vi "Define Sweep Segments Table.vi"(0 "VISA resource name":refnum<visa-resource-name>, 1 "Stimulus Mode (0: Start/Stop)":u16(ring) items=["Start/Stop", "Center/Span"], 2 "Number of Segments (1)":i32=1, 3 "Start/Center (0)":dbl[](array[numeric]), 4 "Stop/Span (0)":dbl[](array[numeric]), 5 "error in (no error)":errorcluster, 6 "Channel (1)":i32=1, 7 "Measurement Points (0)":dbl[](array[numeric]), 8 "Sweep Mode  (0)":dbl[](array[numeric]), 9 "IF Bandwidth (0)":dbl[](array[numeric]), 10 "Sweep Time (F: Disable)":bool, 11 "Power  (0)":dbl[](array[numeric]), 12 "Sweep Time  (0)":dbl[](array[numeric]), 13 "Sweep Delay Time  (0)":dbl[](array[numeric])) -> (14 "VISA resource name out":refnum<visa-resource-name>, 19 "error out":errorcluster)   [LabVIEW 2018, in "Agilent ENA Series.lvlib"]
doc: "Loads the sweep segments into instrument."
uses:
  Agilent ENA Series.lvlib
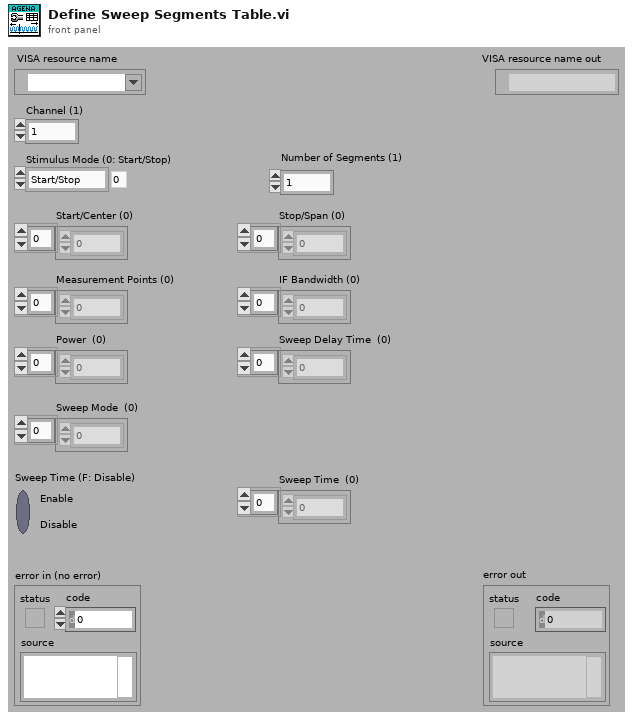
[diagram p1: front panel]
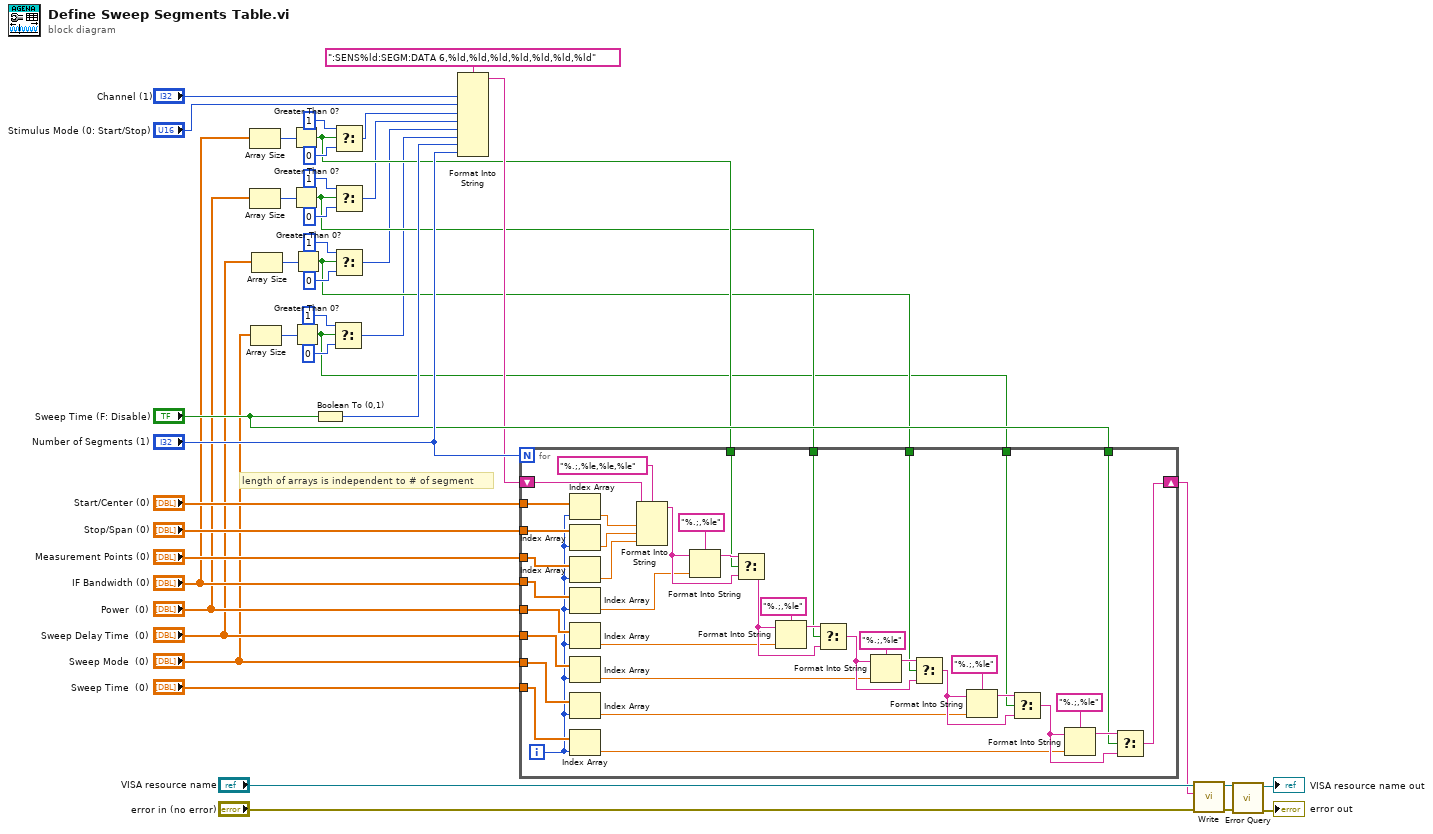
[diagram p0: block diagram]
diagram:
  # "length of arrays is independent to # of segment"
  n1 = Array Size(array="IF Bandwidth (0)") -> (size(s)=w21:i32)
  n2 = Array Size(array="Power  (0)") -> (size(s)=w18:i32)
  n3 = Array Size(array="Sweep Mode  (0)") -> (size(s)=w6:i32)
  n4 = Array Size(array="Sweep Delay Time  (0)") -> (size(s)=w10:i32)
  n5 = Greater Than 0?(x=w21) -> (x > 0?=w20:bool)
  n6 = Greater Than 0?(x=w18) -> (x > 0?=w15:bool)
  n7 = Greater Than 0?(x=w6) -> (x > 0?=w2:bool)
  n8 = Greater Than 0?(x=w10) -> (x > 0?=w9:bool)
  n9 = Boolean To (0,1)(Boolean="Sweep Time (F: Disable)") -> (0, 1=w37:i16)
  n10 = Select(t=1, s=w2, f=0) -> (s? t:f=w3:i32)
  n11 = Select(t=1, s=w20, f=0) -> (s? t:f=w19:i32)
  n12 = Select(t=1, s=w15, f=0) -> (s? t:f=w14:i32)
  n13 = Select(t=1, s=w9, f=0) -> (s? t:f=w8:i32)
  n14 = Format Into String(format string=":SENS%ld:SEGM:DATA 6,%ld,%ld,%ld,%ld,%ld,%ld,%ld", "Channel (1)", "Stimulus Mode (0: Start/Stop)", w19, w14, w8, w3, w37, "Number of Segments (1)") -> (resulting string=w30:string)  [unwired: 2 in, 1 out]
  n15 = for {
    N: "Number of Segments (1)" -> [_]
    tunnel: "Start/Center (0)" -> [w45]
    tunnel: "Stop/Span (0)" -> [w47]
    tunnel: "Measurement Points (0)" -> [w48]
    tunnel: w20 -> [w78]
    tunnel: "IF Bandwidth (0)" -> [w50]
    tunnel: w15 -> [w74]
    tunnel: "Sweep Delay Time  (0)" -> [w55]
    tunnel: w9 -> [w70]
    tunnel: "Sweep Mode  (0)" -> [w57]
    tunnel: w2 -> [w66]
    tunnel: "Sweep Time (F: Disable)" -> [w62]
    shift-right: [w60] -> w29
    shift-left: w30 -> [w61]
    tunnel: "Sweep Time  (0)" -> [w59]
    tunnel: "Power  (0)" -> [w53]
    i -> [w43]
    n16 = Index Array(array=w45, index=w43) -> (element=w46:dbl)
    n17 = Index Array(array=w47, index=w43) -> (element=w44:dbl)
    n18 = Index Array(array=w48, index=w43) -> (element=w49:dbl)
    n19 = Index Array(array=w50, index=w43) -> (element=w51:dbl)
    n20 = Index Array(array=w53, index=w43) -> (element=w52:dbl)
    n21 = Index Array(array=w55, index=w43) -> (element=w54:dbl)
    n22 = Index Array(array=w57, index=w43) -> (element=w56:dbl)
    n23 = Index Array(array=w59, index=w43) -> (element=w58:dbl)
    n24 = Format Into String(format string="%.;,%le,%le,%le", initial string=w61, w46, w44, w49) -> (resulting string=w79:string)  [unwired: 1 in, 1 out]
    n25 = Format Into String(format string="%.;,%le", initial string=w79, w51) -> (resulting string=w80:string)  [unwired: 1 in, 1 out]
    n26 = Select(t=w80, s=w78, f=w79) -> (s? t:f=w75:string)
    n27 = Format Into String(format string="%.;,%le", initial string=w75, w52) -> (resulting string=w77:string)  [unwired: 1 in, 1 out]
    n28 = Select(t=w77, s=w74, f=w75) -> (s? t:f=w71:string)
    n29 = Format Into String(format string="%.;,%le", initial string=w71, w54) -> (resulting string=w72:string)  [unwired: 1 in, 1 out]
    n30 = Select(t=w72, s=w70, f=w71) -> (s? t:f=w67:string)
    n31 = Format Into String(format string="%.;,%le", initial string=w67, w56) -> (resulting string=w69:string)  [unwired: 1 in, 1 out]
    n32 = Select(t=w69, s=w66, f=w67) -> (s? t:f=w63:string)
    n33 = Format Into String(format string="%.;,%le", initial string=w63, w58) -> (resulting string=w64:string)  [unwired: 1 in, 1 out]
    n34 = Select(t=w64, s=w62, f=w63) -> (s? t:f=w60:string)
  }
  n35 = call "Write.vi"("error in (no error)"="error in (no error)", "String ()"=w29, "VISA resource name"="VISA resource name") -> ("error out"=w27:errorcluster, "VISA resource name out"=w28:refnum<visa-resource-name>)  [unwired: 6 in, 1 out]
  n36 = call "Error Query.vi"("error in (no error)"=w27, "VISA resource name"=w28) -> ("error out"=→"error out":errorcluster, "VISA resource name out"=→"VISA resource name out":refnum<visa-resource-name>)  [unwired: 6 in, 2 out]
